vi "Get E&S message from emibin file.vi"(0 "refnum in":refnum<file>, 11 "error in (no error)":errorcluster) -> (4 "refnum out":refnum<file>, 15 "error out":errorcluster)   [LabVIEW 2011]
uses:
  emi Lib/System 01/0 - General/S&E reporting/Private/_emi_ S&E Message.ctl
  emi Lib/System 01/0 - General/S&E reporting/Private/_emi_ S&E Message type.ctl
panel:
  out "EOF":bool
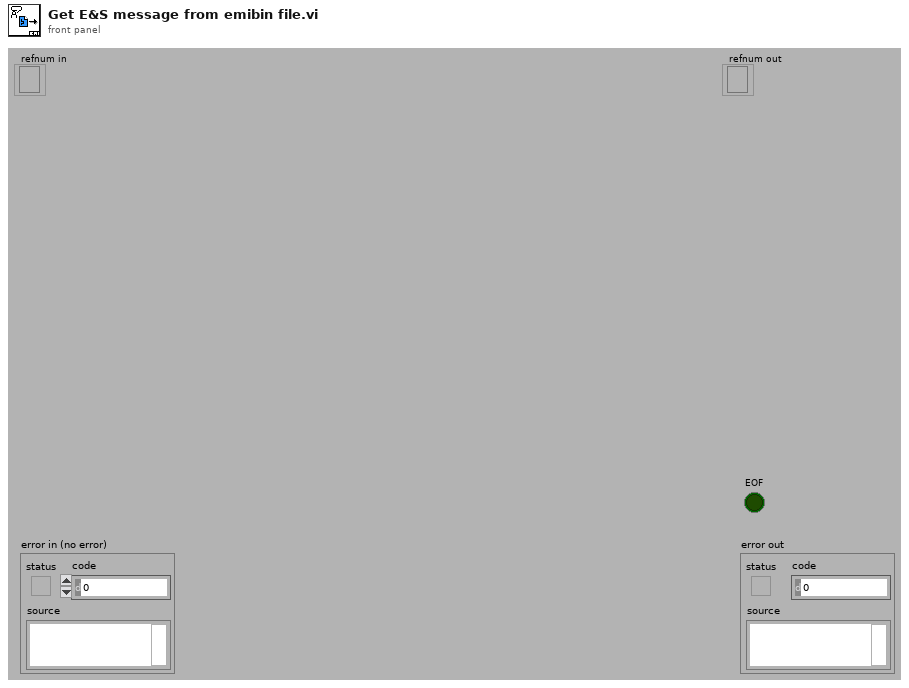
[diagram p1: front panel]
types:
  T1 = typedef "_emi_ S&E Message.ctl" = cluster{"Type":T2, "Originate time":dbl, "System":u8, "Loop":u16, "Sub ID":u16, "Elevated priority":bool, "E&S Message content":variant}
  T2 = typedef "_emi_ S&E Message type.ctl" = enum16{"Error/Warning", "Note", "Debug", "Event", "Alarm Analog", "Alarm Digital", "Annotation"}
  T3 = enum16{"big-endian, network order", "native, host order", "little-endian"}
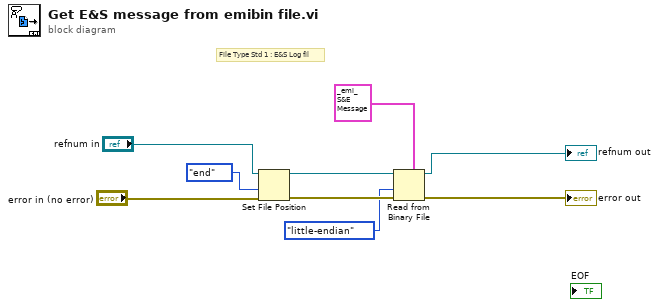
[diagram p0: block diagram]
diagram:
  # "File Type Std 1 : E&S Log fil"
  n1 = Set File Position(refnum="refnum in", from (0:start)=enum16{"start", "end", "current"}."end", error in="error in (no error)") -> (refnum out=w5:refnum<file>, error out=w6:errorcluster)  [unwired: 1 in]
  n2 = Read from Binary File(5:T1 {"Type"=enum."Error/Warning", "Originate time"=nan, "System"=0, "Loop"=9999, "Sub ID"=0, "Elevated priority"=FALSE, "E&S Message content"=variant} ("E&S Message"), 8:w6, 9:T3."little-endian" ("byte order (0:big-endian, network order)"), 11:w5) -> (0:→"error out":errorcluster, 3:→"refnum out":refnum<file>)  [unwired: 2 in, 2 out]
